vi "Power Off.vi"(8 "error in (no error)":errorcluster, 11 "FunctionGenerator in":refnum<class "FunctionGenerator.lvclass">) -> (0 "error out":errorcluster, 3 "FunctionGenerator out":refnum<class "FunctionGenerator.lvclass">)   [LabVIEW 2019, in "FunctionGenerator.lvlib" / "FunctionGenerator.lvclass"]
uses:
  Library/FunctionGenerator.lvclass
  Library/FunctionGenerator.lvclass/FunctionGenerator.ctl
  builds/Instruments/Instruments.lvlibp/Library/Instruments.lvclass
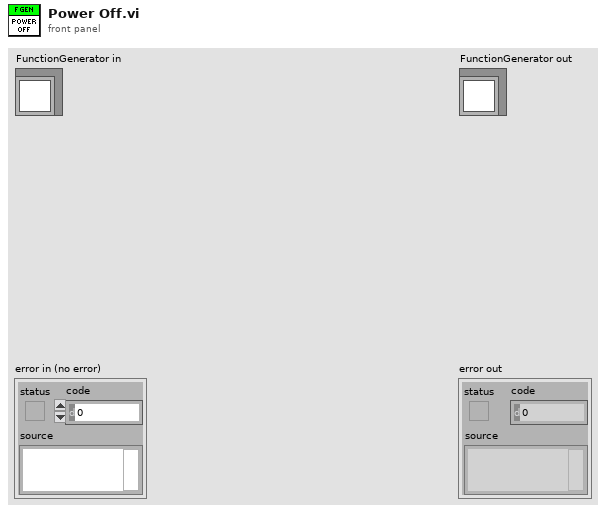
[diagram p1: front panel]
types:
  T1 = typedef "FunctionGenerator.lvlib/FunctionGenerator.lvclass/WaveformSettings.ctl" = cluster{"Frequency":dbl, "Amplitude":dbl, "Offset":dbl, "Phase":dbl, "Symmetry":dbl, "Pulse Width":dbl, "Rise Time":dbl, "Fall Time":dbl, "Mode":T2, "Termination":enum16{"50_Ohm", "High_Z"}, "Output":bool}
  T2 = typedef "FunctionGenerator.lvlib/FunctionGenerator.lvclass/WaveformMode.ctl" = enum16{"Sine", "Square", "Ramp", "Pulse", "Arbitrary", "Triangle", "Noise", "DC"}
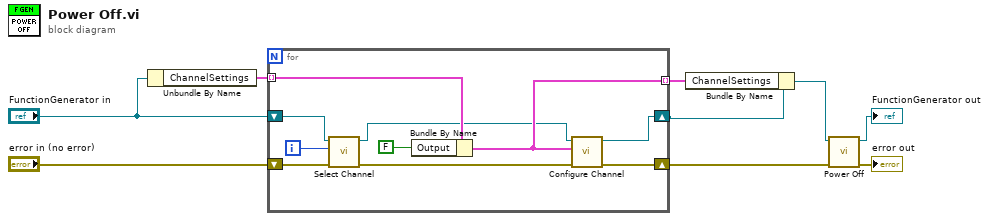
[diagram p0: block diagram]
diagram:
  n1 = Unbundle By Name("FunctionGenerator in") -> ("ChannelSettings"=w7:T1[])
  n2 = for {
    tunnel: w7 -> [w17] mode=indexing
    shift-right: [w19] -> w4
    shift-left: "error in (no error)" -> [w14]
    shift-right: [w18] -> w3
    shift-left: "FunctionGenerator in" -> [w12]
    tunnel: [w15] -> w2 mode=indexing
    i -> [w10]
    n3 = call "Select Channel.vi"("error in (no error)"=w14, "Active Channel"=w10, "FunctionGenerator in"=w12) -> ("error out"=w13:errorcluster, "FunctionGenerator out"=w11:refnum<class "FunctionGenerator.lvclass">)  [unwired: 7 in]
    n4 = Bundle By Name(cluster=w17, "Output"=FALSE) -> (w15:T1)
    n5 = call-dynamic "Configure Channel.vi"("error in (no error)"=w13, "Settings"=w15, "FunctionGenerator in"=w11) -> ("error out"=w19:errorcluster, "FunctionGenerator out"=w18:refnum<class "FunctionGenerator.lvclass">)  [unwired: 7 in]
  }
  n6 = Bundle By Name(cluster=w3, "ChannelSettings"=w2) -> (w1:refnum<class "FunctionGenerator.lvclass">)
  n7 = call-parent "Power Off.vi"("error in (no error)"=w4, "Instruments in"=w1) -> ("error out"=→"error out":errorcluster, "Instruments out"=→"FunctionGenerator out":refnum<class "FunctionGenerator.lvclass">)  [unwired: 8 in]
